vi "Negate_Qin_4chan.vi"(4 "DC offset chan 3":fxp<+/-,32,14>, 6 "DC offset chan 2":fxp<+/-,32,14>, 8 "valid in":bool, 9 "DC offset chan 1":fxp<+/-,32,14>, 10 "DC offset chan 0":fxp<+/-,32,14>, 11 "Data in":fxp<+/-,32,14>[](array[numeric])=[0.0, 0.0, 0.0, 0.0, 0.0, 0.0, 0.0, 0.0]) -> (0 "valid out":bool, 3 "Data out":fxp<+/-,32,14>[](array[numeric]))   [LabVIEW 2018]
uses:
  <vilib>/rvi/FXPMathLib/FxpSub/XNode/nifxpmath_Sub.xnode
  <vilib>/rvi/FXPMathLib/sim/FxpSim.dll
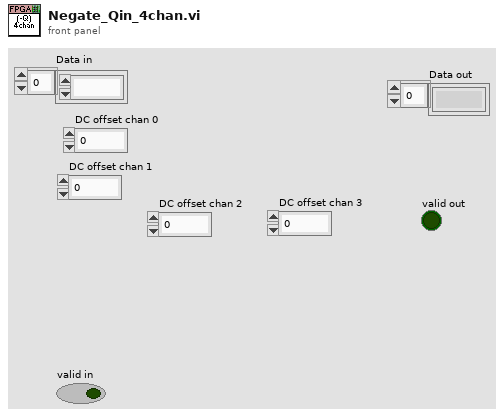
[diagram p1: front panel]
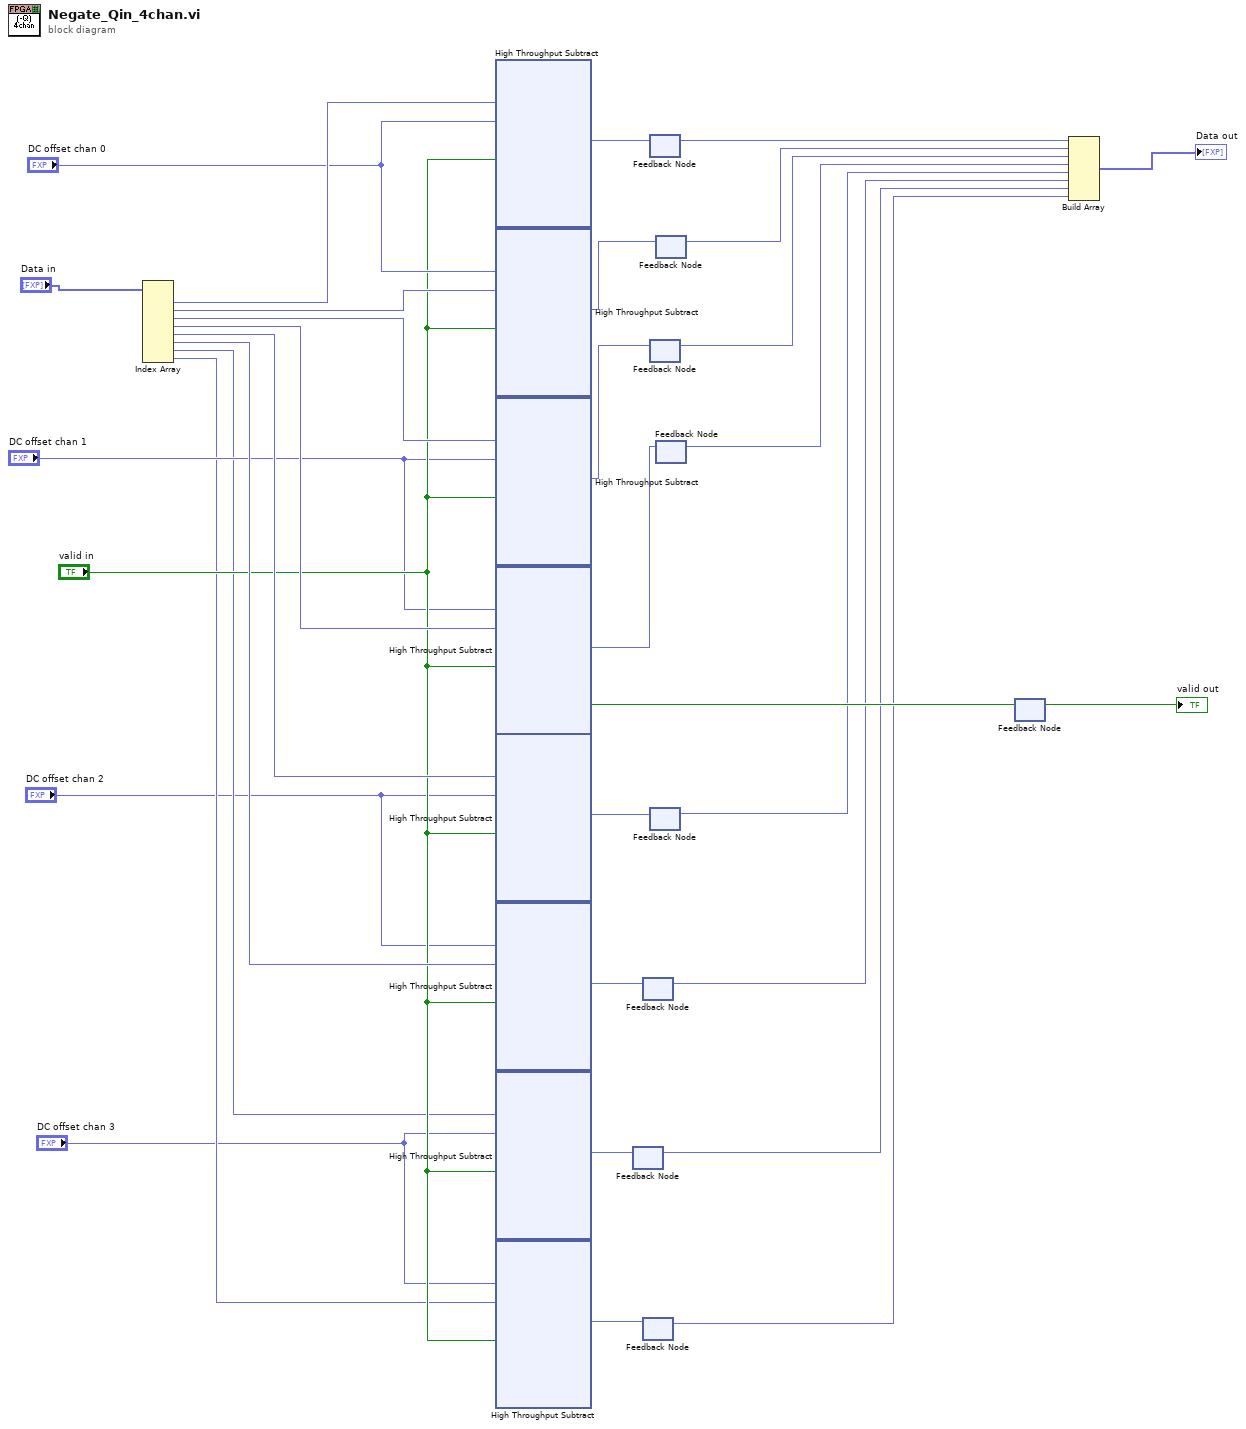
[diagram p0: block diagram]
diagram:
  n1 = Index Array(array="Data in") -> (element #1=w28:fxp<+/-,32,14>, element #2=w27:fxp<+/-,32,14>, element #3=w26:fxp<+/-,32,14>, element #4=w25:fxp<+/-,32,14>, element #5=w16:fxp<+/-,32,14>, element #6=w15:fxp<+/-,32,14>, element #7=w12:fxp<+/-,32,14>, element #8=w11:fxp<+/-,32,14>)  [unwired: 8 in]
  n2 = xnode "High Throughput Subtract"("x"=w28, "y"="DC offset chan 0", "input valid"="valid in") -> ("x-y"=w30:fxp<+/-,32,14>)  [unwired: 1 in, 2 out]
  n3 = xnode "High Throughput Subtract"("x"="DC offset chan 0", "y"=w27, "input valid"="valid in") -> ("x-y"=w23:fxp<+/-,32,14>)  [unwired: 1 in, 2 out]
  n4 = xnode "High Throughput Subtract"("x"=w26, "y"="DC offset chan 1", "input valid"="valid in") -> ("x-y"=w29:fxp<+/-,32,14>)  [unwired: 1 in, 2 out]
  n5 = xnode "High Throughput Subtract"("x"="DC offset chan 1", "y"=w25, "input valid"="valid in") -> ("x-y"=w24:fxp<+/-,32,14>, "output valid"=w18:bool)  [unwired: 1 in, 1 out]
  n6 = xnode "High Throughput Subtract"("x"=w16, "y"="DC offset chan 2", "input valid"="valid in") -> ("x-y"=w10:fxp<+/-,32,14>)  [unwired: 1 in, 2 out]
  n7 = xnode "High Throughput Subtract"("x"="DC offset chan 2", "y"=w15, "input valid"="valid in") -> ("x-y"=w9:fxp<+/-,32,14>)  [unwired: 1 in, 2 out]
  n8 = xnode "High Throughput Subtract"("x"=w12, "y"="DC offset chan 3", "input valid"="valid in") -> ("x-y"=w7:fxp<+/-,32,14>)  [unwired: 1 in, 2 out]
  n9 = xnode "High Throughput Subtract"("x"="DC offset chan 3", "y"=w11, "input valid"="valid in") -> ("x-y"=w8:fxp<+/-,32,14>)  [unwired: 1 in, 2 out]
  n10 = feedback #1() -> (w4:fxp<+/-,32,14>)  [unwired: 1 in]
  n11 = feedback-in #1(w7) -> ()
  n12 = feedback #2() -> (w5:fxp<+/-,32,14>)  [unwired: 1 in]
  n13 = feedback-in #2(w9) -> ()
  n14 = feedback #3() -> (w3:fxp<+/-,32,14>)  [unwired: 1 in]
  n15 = feedback-in #3(w8) -> ()
  n16 = feedback #4() -> (w22:fxp<+/-,32,14>)  [unwired: 1 in]
  n17 = feedback-in #4(w30) -> ()
  n18 = feedback #5() -> (w20:fxp<+/-,32,14>)  [unwired: 1 in]
  n19 = feedback-in #5(w29) -> ()
  n20 = feedback #6() -> (w6:fxp<+/-,32,14>)  [unwired: 1 in]
  n21 = feedback-in #6(w10) -> ()
  n22 = feedback #7() -> (w21:fxp<+/-,32,14>)  [unwired: 1 in]
  n23 = feedback-in #7(w23) -> ()
  n24 = feedback #8() -> (w19:fxp<+/-,32,14>)  [unwired: 1 in]
  n25 = feedback-in #8(w24) -> ()
  n26 = feedback #9() -> (→"valid out":bool)  [unwired: 1 in]
  n27 = feedback-in #9(w18) -> ()
  n28 = Build Array(w22, w21, w20, w19, w6, w5, w4, w3) -> (→"Data out":fxp<+/-,32,14>[])
